vi "DataCalibrater.vi"(2 "CalCoefficients":fxp<+/-,33,14>[](array[numeric])=[0.0, 0.0, 0.0, 0.0], 7 "RawData":fxp<+/-,33,14> format="%#_24g") -> (8 "DataOut":fxp<+/-,33,14> format="%#_24g")   [LabVIEW 2013]
uses:
  <vilib>/rvi/FXPMathLib/FxpMul/XNode/nifxpmath_Multiplier.xnode
  <vilib>/rvi/FXPMathLib/FxpAdd/XNode/nifxpmath_Add.xnode
  <vilib>/rvi/FXPMathLib/sim/FxpSim.dll
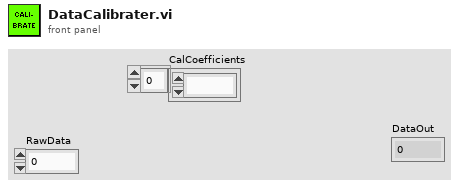
[diagram p1: front panel]
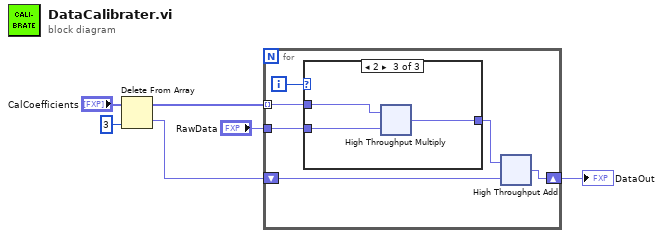
[diagram p0: block diagram]
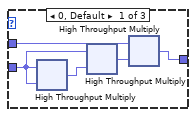
[diagram p2: hidden frame]
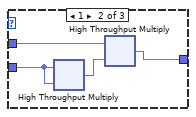
[diagram p3: hidden frame]
diagram:
  n1 = Delete From Array(array="CalCoefficients", index=3) -> (deleted portion=w2:fxp<+/-,33,14>, array with subset deleted=w6:fxp<+/-,33,14>[])  [unwired: 1 in]
  n2 = for {
    tunnel: w6 -> [w11] mode=indexing
    tunnel: "RawData" -> [w10]
    shift-right: [w7] -> w1
    shift-left: w2 -> [w8]
    i -> [w12]
    n3 = case shown="2" w12 {
      tunnel: w11 -> [w17 w21 w24]
      tunnel: w10 -> [w16 w20 w23]
      tunnel: [w13 w18 w22] -> w9
      frame 0, Default {
        n4 = xnode "High Throughput Multiply"("x"=w16, "y"=w16) -> ("x*y"=w15:fxp<+/-,33,14>)
        n5 = xnode "High Throughput Multiply"("x"=w16, "y"=w15) -> ("x*y"=w14:fxp<+/-,33,14>)
        n6 = xnode "High Throughput Multiply"("x"=w17, "y"=w14) -> ("x*y"=w13:fxp<+/-,33,14>)
      }
      frame 1 {
        n7 = xnode "High Throughput Multiply"("x"=w20, "y"=w20) -> ("x*y"=w19:fxp<+/-,33,14>)
        n8 = xnode "High Throughput Multiply"("x"=w21, "y"=w19) -> ("x*y"=w18:fxp<+/-,33,14>)
      }
      frame 2 {
        n9 = xnode "High Throughput Multiply"("x"=w24, "y"=w23) -> ("x*y"=w22:fxp<+/-,33,14>)
      }
    }
    n10 = xnode "High Throughput Add"("x"=w9, "y"=w8) -> ("x+y"=w7:fxp<+/-,33,14>)
  }
  "DataOut" <- w1
